vi "Light-Sensor.vi"() -> ()   [LabVIEW 2016, in "EV3Group10.lvrbt"]
uses:
  EV3Group10.lvrbt
  <vilib>/NXT/Block Support/NXT_InputPort.ctl
  <vilib>/NXT/Block Support/NXT_OutputPort.ctl
  <vilib>/NXT/Dual Mode Library/Waits/Wait_Touch.vi
  <vilib>/NXT/Dual Mode Library/Waits/Wait_Num.vi
  <vilib>/NXT/Dual Mode Library/Sensors/EV3_Color_Reflect.vi
  <vilib>/NXT/NXTIO Xnodes/NXTIONodeSubVIs/NXTMoveMotors.vi
  <vilib>/NXT/NXTIO Xnodes/NXTIONodeSubVIs/NXTStopMotors.vi
  <vilib>/NXT/NXTIO Xnodes/AddressXNode/NXTIOAddress.xnode
  <vilib>/NXT/NXTIO Xnodes/NXTIOXNode/NXTIO.xnode
  <vilib>/NXT/Subs/LVHSConnector.ctl
  <vilib>/NXT/Dual Mode Library/Display/drawText.vi
  <vilib>/NXT/LegoClasses/BrickReference/BrickReference.lvclass
panel:
  out "Signal 2":dbl
  out "Signal 1":dbl
  out "Average Signal":dbl
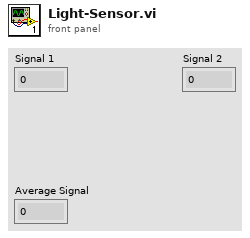
[diagram p1: front panel]
types:
  T1 = typedef "NXT_InputPort.ctl" = u32
  T2 = typedef "LVHSConnector.ctl" = refnum<class "BrickReference.lvclass">
  T3 = typedef "NXT_OutputPort.ctl" = u8
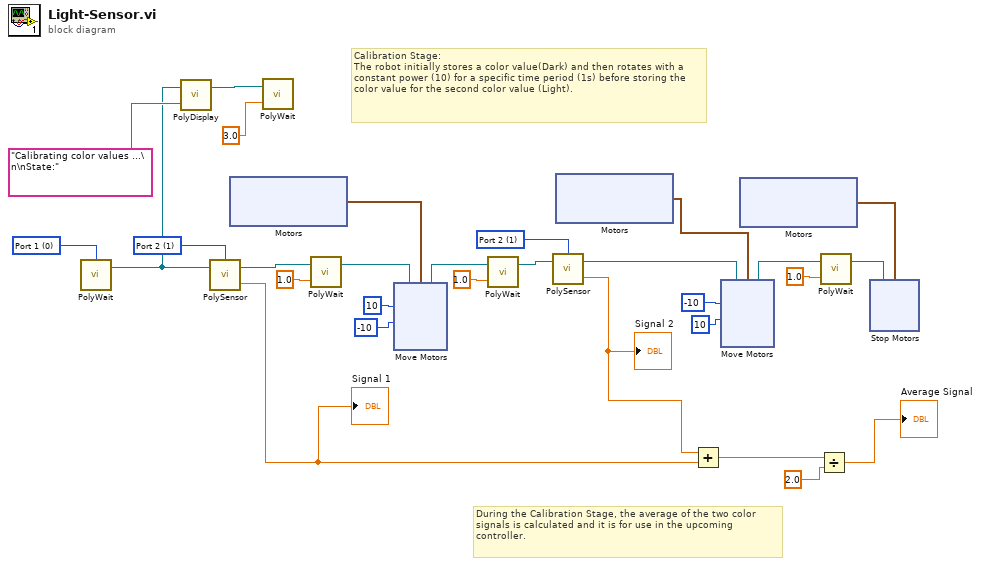
[diagram p0: block diagram]
diagram:
  w10 = T1 1 items=["Port 1", "Port 2", "Port 3", "Port 4"] ("Port (Port 1)")
  w15 = T1 0 items=["Port 1", "Port 2", "Port 3", "Port 4"] ("Port (Port 1)")
  w29 = T1 1 items=["Port 1", "Port 2", "Port 3", "Port 4"] ("Port (Port 1)")
  # "During the Calibration Stage, the average of the two color signals is calculated and it is for use in the upcoming controller."
  # "Calibration Stage:\nThe robot initially stores a color value(Dark) and then rotates with a constant power (10) for a specific time period (1s) before storing the color value for the second color value (Light)."
  n1 = call-poly <vilib>:"PolyWait.vi"("Port (Port 1)"=w15) -> ("NXT/EV3"=w7:T2)  [unwired: 3 in]
  n2 = call-poly <vilib>:"PolyDisplay.vi"("Text"="Calibrating color values ...\n\nState:", "NXT/EV3"=w7) -> ("NXT/EV3"=w17:T2)  [unwired: 2 in]
  n3 = call-poly <vilib>:"PolySensor.vi"("NXT/EV3"=w7, "Port (Port 1)"=w10) -> ("Scaled Value"=w2:sgl, "NXT/EV3"=w9:T2)  [unwired: 1 in]
  "Signal 1" <- w2
  n4 = xnode "Motors"() -> ("Motor"=w28:cluster{"Port":T3, "Port":T3})
  n5 = call-poly <vilib>:"PolyWait.vi"("Time (1 sec)"=sgl 3.0, "NXT/EV3"=w17) -> ()  [unwired: 2 in, 1 out]
  n6 = call-poly <vilib>:"PolyWait.vi"("Time (1 sec)"=sgl 1.0, "NXT/EV3"=w9) -> ("NXT/EV3"=w11:T2)  [unwired: 2 in]
  n7 = xnode "Move Motors"("Power/Speed 2"=i8 -10, "Power/Speed 1"=i8 10, "Motors"=w28, "NXT/EV3"=w11) -> ("NXT/EV3"=w18:T2)
  n8 = call-poly <vilib>:"PolyWait.vi"("Time (1 sec)"=sgl 1.0, "NXT/EV3"=w18) -> ("NXT/EV3"=w14:T2)  [unwired: 2 in]
  n9 = call-poly <vilib>:"PolySensor.vi"("NXT/EV3"=w14, "Port (Port 1)"=w29) -> ("Scaled Value"=w1:sgl, "NXT/EV3"=w13:T2)  [unwired: 1 in]
  "Signal 2" <- w1
  n10 = xnode "Motors"() -> ("Motor"=w24:cluster{"Port":T3, "Port":T3})
  n11 = Add(x=w1, y=w2) -> (x+y=w6:sgl)
  n12 = xnode "Move Motors"("Power/Speed 2"=i8 10, "Power/Speed 1"=i8 -10, "Motors"=w24, "NXT/EV3"=w13) -> ("NXT/EV3"=w21:T2)
  n13 = xnode "Motors"() -> ("Motor"=w4:cluster{"Port":T3, "Port":T3})
  n14 = Divide(x=w6, y=sgl 2.0) -> (x/y=→"Average Signal":sgl)
  n15 = call-poly <vilib>:"PolyWait.vi"("Time (1 sec)"=sgl 1.0, "NXT/EV3"=w21) -> ("NXT/EV3"=w8:T2)  [unwired: 2 in]
  n16 = xnode "Stop Motors"("Motors"=w4, "NXT/EV3"=w8) -> ()  [unwired: 1 out]
